vi "Add Panel Tier.vi"(8 "Error In":errorcluster, 9 "Old VI's Destination":refnum<class "Panel.lvclass"> caption="Replaced Tier's Panel (no panel)", 10 "New VI Ref":refnum<vi> caption="New VI Ref (caller)", 11 "Panel Actor in":refnum<class "Panel Actor.lvclass">) -> (0 "Error Out":errorcluster, 1 "Replaced VI":string, 3 "Panel Actor out":refnum<class "Panel Actor.lvclass">)   [LabVIEW 2017, in "MGI-Panel Actor.lvlib" / "Panel Actor.lvclass"]
doc: "Adds a new Tier to the panel. Use Panel Tiers to dynamically build UIs that reflect the inheritance of the actor.\n\nWire a VI into <b>New VI Ref</b> to replace VI with a different one.\n\nWire <b>Replaced Tier's Panel</b> to insert the replaced VI in another panel.\n\nThis is useful when creating dynamic UIs that have layers at each chain in the override list. Each parent can use this VI to insert themselves at the base tier, and insert the last layer in a subpanel, for example.\n\nSee the \"Tiered Panel\" example for more information.\n\n<B>Panel Actor In:</B> Panel Actor object.\n<B>New VI Ref:</B> VI reference for the new vi.\n<B>Replaced Tier's Panel:</B> Panel object for the replaced tier.\n<B>Error In:</B> Describes error conditions that occur before this node runs.\n\n<B>Panel Actor Out:</B> Panel Actor object.\n<B>Error Out:</B> Contains error information.\n----\nCopyright: MGI 2018\nAuthor: Derek Trepanier"
uses:
  Panel Actor.lvclass
  panel-manager/Source/Panel/Panel.lvclass
  Panel Actor.lvclass/Panel Actor.ctl
  <vilib>/Utility/error.llb/Error Cluster From Error Code.vi
  <vilib>/ErrorRing/Error Ring.xnode
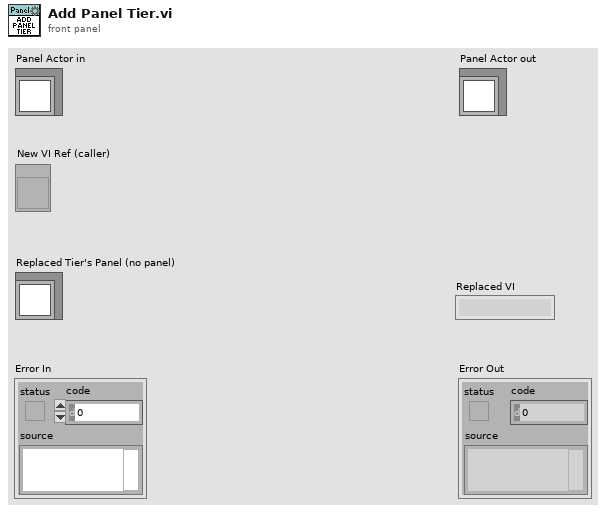
[diagram p1: front panel]
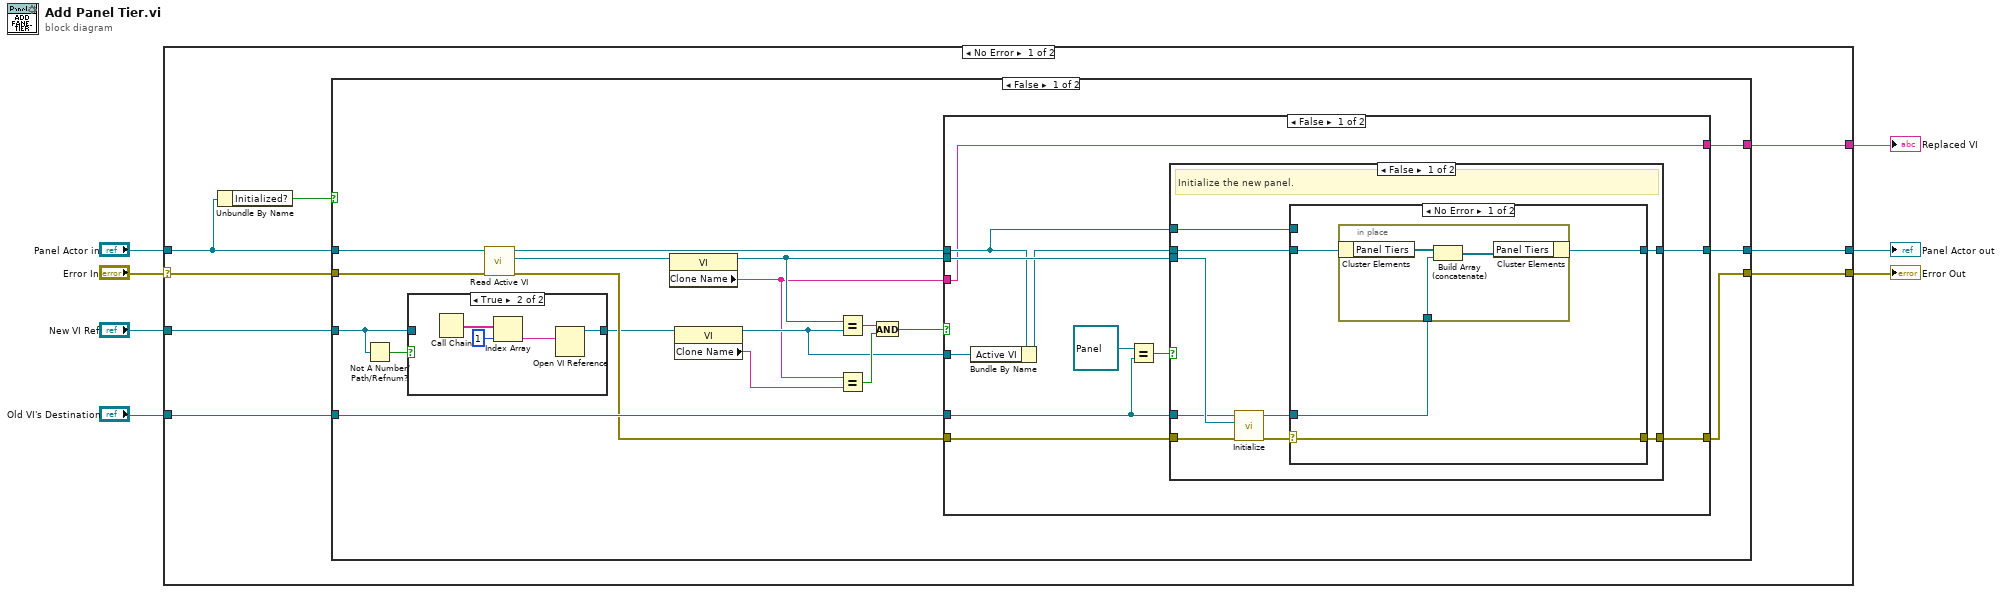
[diagram p0: block diagram]
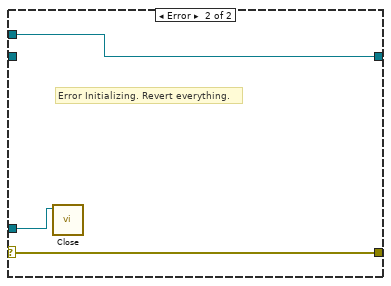
[diagram p3: hidden frame]
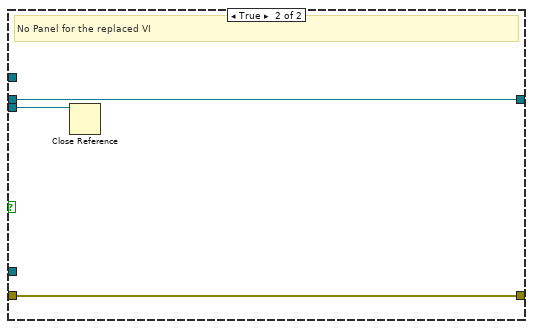
[diagram p4: hidden frame]
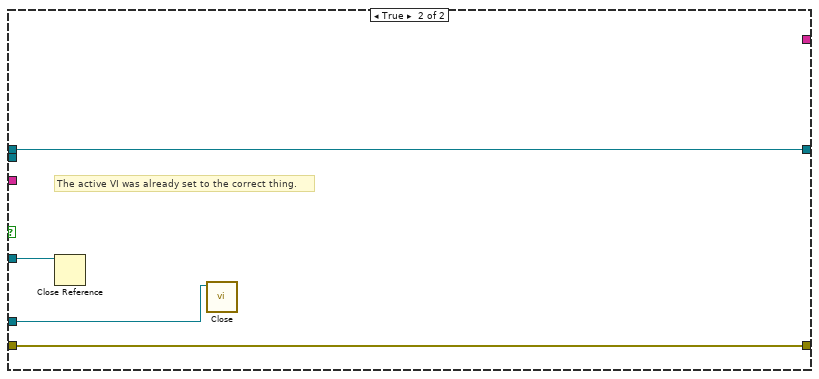
[diagram p5: hidden frame]
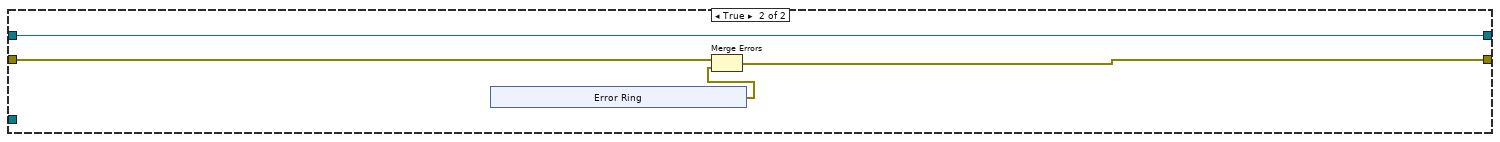
[diagram p6: hidden frame]
diagram:
  n1 = case shown="No Error" "Error In" {
    selector: "Error In" -> [w15 w87]
    tunnel: [w12 w87] -> w6
    tunnel: [w11 w86] -> w4
    tunnel: "Panel Actor in" -> [w10 w86]
    tunnel: "New VI Ref" -> [w13 _]
    tunnel: "Old VI's Destination" -> [w14 _]
    tunnel: [w8 _] -> w1
    frame No Error {
      n2 = Unbundle By Name(w10) -> ("Initialized?"=w9:bool)
      n3 = case shown="False" w9 {
        tunnel: w15 -> [w33 w79]
        tunnel: w14 -> [w32 _]
        tunnel: w13 -> [w29 _]
        tunnel: [w20 w78] -> w12
        tunnel: w10 -> [w19 w80]
        tunnel: [w18 w80] -> w11
        tunnel: [w16 _] -> w8
        frame False {
          n4 = Not A Number/Path/Refnum?(number/path/refnum=w29) -> (NaN/Path/Refnum?=w30:bool)
          n5 = case shown="True" w30 {
            tunnel: w29 -> [w35 _]
            tunnel: [w35 w36] -> w25
            frame False {
            }
            frame True {
              n6 = Call Chain() -> (call chain=w39:string[])
              n7 = Index Array(array=w39, index=1) -> (element=w37:string)
              n8 = Open VI Reference(vi path=w37) -> (vi reference=w36:refnum<vi>)  [unwired: 5 in, 1 out]
            }
          }
          n9 = call "Read Active VI.vi"("error in (no error)"=w33, "Panel Actor in"=w19) -> ("error out"=w31:errorcluster, "Active VI ref"=w26:refnum<vi>, "Panel Actor out"=w34:refnum<class "Panel Actor.lvclass">)  [unwired: 7 in]
          n10 = property class="VI"(reference=w26) -> (reference out=w21:refnum<vi>, "Clone Name"=w17:string)  [unwired: 1 in, 1 out]
          n11 = property class="VI"(reference=w25) -> (reference out=w22:refnum<vi>, "Clone Name"=w24:string)  [unwired: 1 in, 1 out]
          n12 = Equal?(x=w21, y=w22) -> (x = y?=w28:bool)
          n13 = Equal?(x=w17, y=w24) -> (x = y?=w23:bool)
          n14 = And(x=w28, y=w23) -> (x .and. y?=w27:bool)
          n15 = case shown="False" w27 {
            tunnel: w32 -> [w44 w73]
            tunnel: w31 -> [w50 w75]
            tunnel: [w49 w75] -> w20
            tunnel: w34 -> [w41 w76]
            tunnel: [w48 w76] -> w18
            tunnel: w22 -> [w45 w74]
            tunnel: w21 -> [w47 _]
            tunnel: w17 -> [w40 _]
            tunnel: [w40 _] -> w16
            frame False {
              n16 = Bundle By Name(cluster=w41, "Active VI"=w45) -> (w46:refnum<class "Panel Actor.lvclass">)
              n17 = Equal?(x=refnum<class "Panel.lvclass"> refnum, y=w44) -> (x = y?=w42:bool)
              n18 = case shown="False" w42 {
                tunnel: w50 -> [w59 w71]
                tunnel: [w52 w71] -> w49
                tunnel: [w58 w72] -> w48
                tunnel: w47 -> [w57 w70]
                tunnel: w46 -> [w56 w72]
                tunnel: w44 -> [w55 _]
                tunnel: w41 -> [w51 _]
                frame False {
                  # "Initialize the new panel."
                  n19 = call "Initialize.vi"("error in (no error)"=w59, "VI Refnum"=w57, "Panel In"=w55) -> ("error out"=w53:errorcluster, "Panel Out"=w54:refnum<class "Panel.lvclass">)  [unwired: 6 in, 1 out]
                  n20 = case shown="No Error" w53 {
                    selector: w53 -> [w60 w67]
                    tunnel: [w63 w69] -> w58
                    tunnel: w56 -> [w62 _]
                    tunnel: w54 -> [w61 w68]
                    tunnel: [w60 w67] -> w52
                    tunnel: w51 -> [_ w69]
                    frame No Error {
                      n21 = in-place {
                        in-place-border: w61 -> [w64]
                        n22 = in-place-cluster #1(w62) -> ("Panel Tiers"=w66:refnum<class "Panel.lvclass">[])
                        n23 = Build Array (concatenate)(w66, w64) -> (w65:refnum<class "Panel.lvclass">[])
                        n24 = in-place-cluster #1("Panel Tiers"=w65) -> (w63:refnum<class "Panel Actor.lvclass">)
                      }
                    }
                    frame Error {
                      # "Error Initializing. Revert everything."
                      n25 = call-dynamic "Close.vi"("Panel In"=w68) -> ()  [unwired: 10 in, 1 out]
                    }
                  }
                }
                frame True {
                  # "No Panel for the replaced VI"
                  n26 = Close Reference(reference=w70) -> ()  [unwired: 1 in, 1 out]
                }
              }
            }
            frame True {
              # "The active VI was already set to the correct thing."
              n27 = Close Reference(reference=w74) -> ()  [unwired: 1 in, 1 out]
              n28 = call-dynamic "Close.vi"("Panel In"=w73) -> ()  [unwired: 10 in, 1 out]
            }
          }
        }
        frame True {
          n29 = xnode "Error Ring"() -> ("error out"=w77:errorcluster)
          n30 = Merge Errors(w79, w77) -> (w78:errorcluster)
        }
      }
    }
    frame Error {
    }
  }
  "Error Out" <- w6
  "Panel Actor out" <- w4
  "Replaced VI" <- w1
